vi "SaveData_Force.vi"(3 "Data Froce":T1, 4 "Name_Test":string(combo)="D_L_", 5 "Lane_Number":string(combo)="ST1_") -> (2 "new file path":path)   [LabVIEW 2017]
uses:
  <vilib>/Utility/file.llb/Read Delimited Spreadsheet (string).vi
  <vilib>/Utility/file.llb/Write Delimited Spreadsheet (string).vi
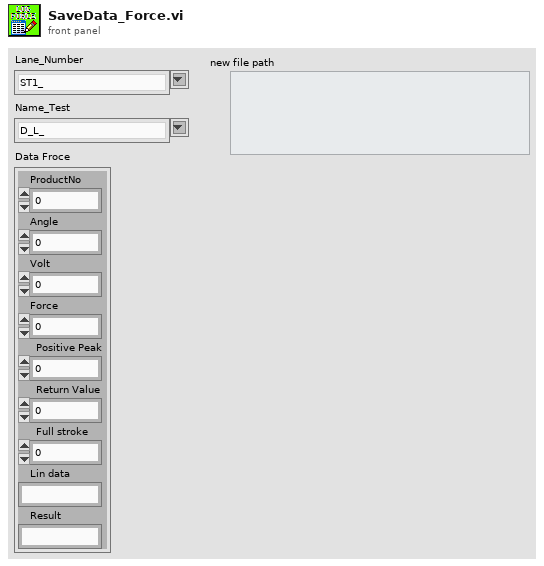
[diagram p1: front panel]
types:
  T1 = cluster{"ProductNo":u16, "Angle":dbl, "Volt":dbl, "Force":dbl, "Positive Peak":dbl, "Return Value":dbl, "Full stroke":dbl, "Lin data":string, "Result":string}
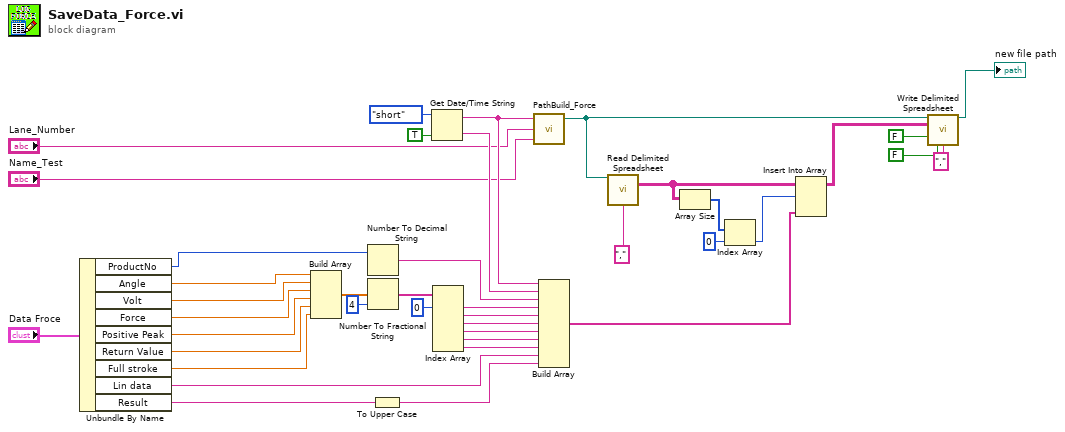
[diagram p0: block diagram]
diagram:
  n1 = Unbundle By Name("Data Froce") -> ("ProductNo"=w14:u16, "Angle"=w22:dbl, "Volt"=w21:dbl, "Force"=w20:dbl, "Positive Peak"=w19:dbl, "Return Value"=w18:dbl, "Full stroke"=w17:dbl, "Lin data"=w16:string, "Result"=w5:string)
  n2 = Build Array(w22, w21, w20, w19, w18, w17) -> (w38:dbl[])
  n3 = Number To Decimal String(number=w14) -> (decimal integer string=w13:string)  [unwired: 1 in]
  n4 = Number To Fractional String(number=w38, precision (6)=i16 4) -> (F-format string=w36:string[])  [unwired: 2 in]
  n5 = To Upper Case(1:w5) -> (0:w4:string)
  n6 = Get Date/Time String(date format (0)=enum16{"short", "long", "abbreviated"}."short", want seconds? (F)=TRUE) -> (date string=w39:string, time string=w34:string)  [unwired: 1 in]
  n7 = Index Array(array=w36, index #1=0 ("index")) -> (element #1=w12:string, element #2=w11:string, element #3=w10:string, element #4=w9:string, element #5=w8:string, element #6=w7:string)  [unwired: 5 in]
  n8 = call "PathBuild_Force.vi"("Name_Test"="Name_Test", "Lane_Number"="Lane_Number", "Date"=w39) -> ("path"=w30:path)  [unwired: 2 in]
  n9 = Build Array "Build Array"(w39, w34, w13, w12, w11, w10, w9, w8, w7, w16, w4) -> (w40:string[])
  n10 = call-poly <vilib>:"Read Delimited Spreadsheet.vi"("file path (dialog if empty)"=w30, "delimiter (\\t)"="," ("delimiter (\\t)")) -> ("all rows"=w28:string[][])  [unwired: 8 in, 5 out]
  n11 = Array Size(array=w28) -> (size(s)=w27:i32[])
  n12 = Index Array(array=w27, index=0) -> (element=w25:i32)
  n13 = Insert Into Array "Insert Into Array"(array=w28, index (row)=w25, new element=w40) -> (w31:string[][])  [unwired: 1 in]
  n14 = call-poly <vilib>:"Write Delimited Spreadsheet.vi"("file path (dialog if empty)"=w30, "2D data"=w31, "append to file? (new file:F)"=FALSE, "transpose? (no:F)"=FALSE, "delimiter (\\t)"="," ("delimiter (\\t)")) -> ("new file path (Not A Path if cancelled)"=→"new file path":path)  [unwired: 9 in, 1 out]
